vi "ResponseStringToSignalCluster(obj).vi"(8 "error in (no error)":errorcluster, 11 "T560Trigger in":refnum<class "T560Trigger.lvclass">) -> (0 "error out":errorcluster, 3 "T560Trigger out":refnum<class "T560Trigger.lvclass">)   [LabVIEW 2020, in "T560Trigger.lvclass"]
doc: "Update the value of 'T560channel.Signal' cluster by converting the 'T560channel.Response' string"
uses:
  T560Trigger.lvclass
  C:/GEECS/Developers Version/source/Device Drivers/Highland T564 DDG/SupportLibraries/DeviceSpecific/HighlandT560Lib/T560ChannelClass/T560Channel.lvclass
  T560Trigger.lvclass/T560Trigger.ctl
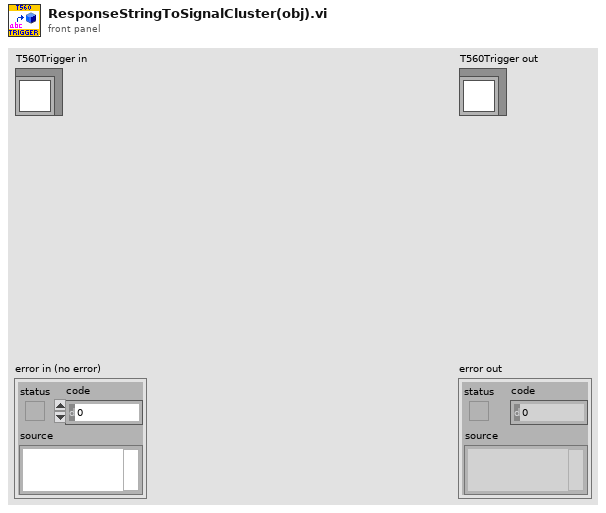
[diagram p1: front panel]
types:
  T1 = typedef "TriggerImpedance.ctl" = enum16{"10KOhm", "50Ohms"}
  T2 = typedef "TriggerSource.ctl" = enum16{"Rising", "Falling", "Internal 80MHz", "Internal DDS", "Remote", "Disabled"}
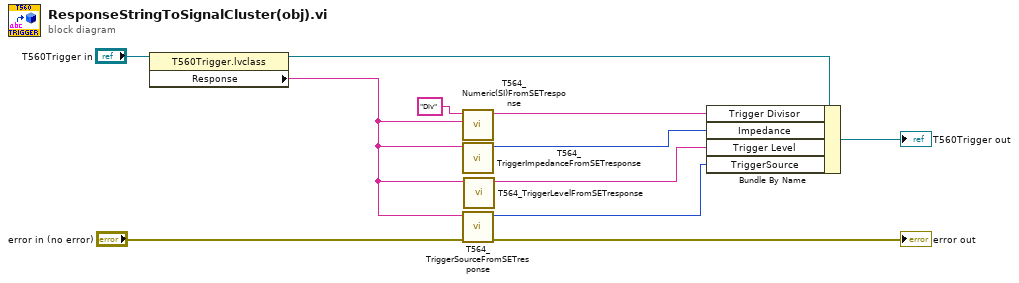
[diagram p0: block diagram]
diagram:
  n1 = property class="T560Trigger.lvclass"(reference="T560Trigger in") -> (reference out=w9:refnum<class "T560Trigger.lvclass">, "Response"=w1:string)  [unwired: 1 in, 1 out]
  n2 = call "T564_Numeric(SI)FromSETresponse.vi"("StringIn"=w1, "Prefix"="Div" ("regular expression")) -> ("SI_String"=w8:string)  [unwired: 9 in]
  n3 = call "T564_TriggerImpedanceFromSETresponse.vi"("String"=w1) -> ("Impedance"=w7:T1)  [unwired: 10 in]
  n4 = call "T564_TriggerSourceFromSETresponse.vi"("error in"="error in (no error)", "String"=w1) -> ("error out"=→"error out":errorcluster, "TriggerSource"=w2:T2)  [unwired: 8 in]
  n5 = call "T564_TriggerLevelFromSETresponse.vi"("StringIn"=w1) -> ("TriggerLevel"=w6:string)  [unwired: 10 in]
  n6 = Bundle By Name(cluster=w9, "Trigger Divisor"=w8, "Impedance"=w7, "Trigger Level"=w6, "TriggerSource"=w2) -> (→"T560Trigger out":refnum<class "T560Trigger.lvclass">)
